vi "Class Property Strings.vi"() -> ()   [LabVIEW 2020, in "Modules.lvlib" / "RSI Module.lvclass"]
uses:
  RSI Module.lvclass
panel:
  in  "Chan #":string="Chan #"
  in  "Module Class":string="Module Class"
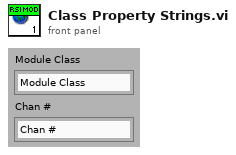
[diagram p1: front panel]
diagram:
